vi "Main.vi"() -> ()   [LabVIEW 2026]
uses:
  3D utilities/3DS Models.ctl
  typedefs/System States.ctl
  typedefs/Render States.ctl
  <vilib>/picture/3D Picture Control/Old 3D Toolkit.llb/model.ctl
  <vilib>/picture/3D Picture Control/Old 3D Toolkit.llb/point3f.ctl
  <vilib>/picture/3D Picture Control/Old 3D Toolkit.llb/VertexMode.ctl
  <vilib>/vision/Image Controls.llb/IMAQ Image.ctl
  XRay Cabinet/XRay Cabinet.lvclass
  C:/Users/Andrey/Desktop/XRaySimulatorLV/XRay Scene/XRay Scene.lvclass
  XRay Beam/XRay Beam.lvclass
  XRay CArm/XRay CArm.lvclass
  XRay Part Sample/XRay Part Sample.lvclass
  XRay Table/XRay Table.lvclass
  XRay Beam/XRay Beam.lvclass/XRay Beam.ctl
  XRay Part Sample/XRay Part Sample.lvclass/XRay Part Sample.ctl
  XRay Table/XRay Table.lvclass/XRay Table.ctl
  <vilib>/Analysis/coordinate.llb/3D Cartesian Coordinate Rotation (Euler) (Scalar).vi
  67ea9b9f-5008-4843-b879-74d7c71b0f0c.vi
  XRay Axis Rails/XRay Axis Rails.lvclass
  <vilib>/picture/3D Picture Control/Object/Create Object.vi
  <vilib>/picture/3D Picture Control/Object/Create Object (name).vi
  <vilib>/picture/3D Picture Control/Geometries/Create 3D Axis.vi
  <vilib>/picture/3D Picture Control/Object/Add Object.vi
  <vilib>/picture/3D Picture Control/Object/Add Object (no reference).vi
  XRay Scene/XRay Scene.lvclass
  <vilib>/vision/NI_Vision_Development_Module.lvlib
  <vilib>/Analysis/NI_AALPro.lvlib
  3D utilities/3D utilities.lvlib
  <vilib>/picture/3D Picture Control/NI_Old 3D Toolkit.lvlib
  LV_3D_Util64.dll
panel:
  in  "Link to Z":bool
  in  "Mode":T1(ring)=enum."Wireframe"
  in  "High Res Render":bool
  in  "Play Button":bool
  in  "Reset":bool
  out "Render":bool
  in  "stop":bool
  in  "Part Angle":dbl(knob) caption="Part\nAngle"
  out "2D Image":T2(plugin-control)
  in  "Model":T3=enum."NI Bottle"
  in  "FDD":sgl(slide)=11.031496 scale=1.0..15.0
  in  "DDA SIZE":sgl(slide)=2.003937 scale=1.0..4.0
  out "Size":i32=1240
  out "Time, ms":dbl=63.153
  out "Max Thickness":sgl=0.5478592
  in  "Y Position":dbl(slide)=7.0 scale=1.0..12.0
  in  "X Position":dbl(slide)=0.5 scale=-2.0..2.0
  in  "C Arm Angle":dbl(knob) caption="C-Arm\nAngle" scale=90.0..-90.0
  in  "Z position":sgl(slide)=4.0 scale=0.0..10.0
  out "3D Picture":refnum<vi>(3d-picture)
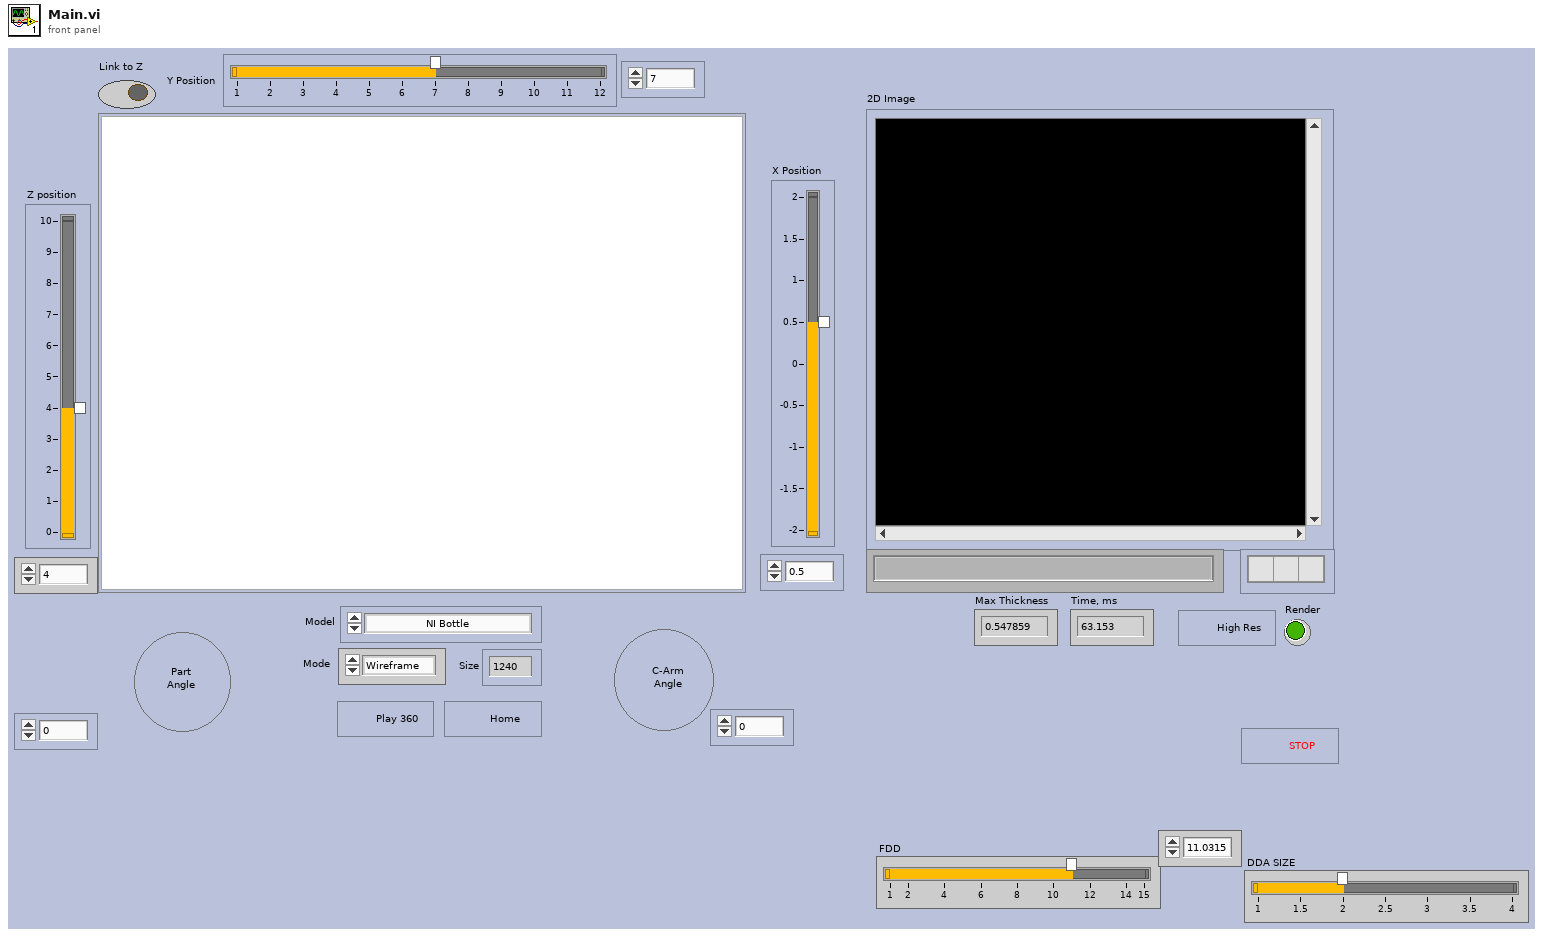
[diagram p1: front panel]
types:
  T1 = enum16{"Inherit Value", "Points", "Wireframe", "Polygons"}
  T2 = typedef "IMAQ Image.ctl" = refnum<image>
  T3 = typedef "3DS Models.ctl" = enum16{"ASTM E2597 Step Wedge", "NI Bottle", "Utah Teapot", "Utah Teapot (Low Res)", "My Cube", "Tree", "Tree 2", "FreeCAD Sample", "Schenkel", "Bunny", "Corona Virus", "Corona Virus (Low Res)", "Offset"}
  T4 = typedef "Render States.ctl" = enum16{"Init", "Create Model", "Move Model", "Render Model", "Render Model (High Res)", "Waiting for Command"}
  T5 = typedef "System States.ctl" = enum16{"Init", "Render", "Waiting for Notification", "Move", "Move 2D Model", "Close and reopen Model", "Quit"}
  T6 = typedef "NI_3D Picture Control.lvlib/NI_Old 3D Toolkit.lvlib/point3f.ctl" = cluster{"x":sgl, "y":sgl, "z":sgl}
  T7 = enum32{"Linear", "Log", "Exp", "Square", "Square root", "Power X", "Power 1/X"}
  T8 = cluster{"XRay Cabinet":refnum<class "XRay Cabinet.lvclass">, "XRay Beam":refnum<class "XRay Beam.lvclass">, "XRay CArm":refnum<class "XRay CArm.lvclass">, "XRay Part Sample":refnum<class "XRay Part Sample.lvclass">, "XRay Table":refnum<class "XRay Table.lvclass">}
  T9 = typedef "Image Type" = u32
  T10 = typedef "NI_3D Picture Control.lvlib/NI_Old 3D Toolkit.lvlib/model.ctl" = cluster{"VertexList":T6[], "FaceList":cluster{"v1":i32, "v2":i32, "v3":i32}[], "NormalList":T6[], "Mode":T11}
  T11 = typedef "NI_3D Picture Control.lvlib/NI_Old 3D Toolkit.lvlib/VertexMode.ctl" = enum16{"GL_POINTS", "GL_LINES", "GL_LINE_LOOP", "GL_LINE_STRIP", "GL_TRIANGLES", "GL_TRIANGLE_STRIP", "GL_TRIANGLE_FAN", "GL_QUADS", "GL_QUAD_STRIP", "GL_POLYGON"}
  T12 = cluster{"Model":T10, "Rendered Image":T2, "Processed Image":T2, "Vertex":T6[], "FaceList":cluster{"v1":i32, "v2":i32, "v3":i32}[]}
  T13 = cluster{"histogram":u32[], "Minimal Value":sgl, "Maximal Value":sgl, "Starting Value":sgl, "Interval Width":sgl, "Mean Value":sgl, "Standard  Variation":sgl, "Area (pixels)":i32}
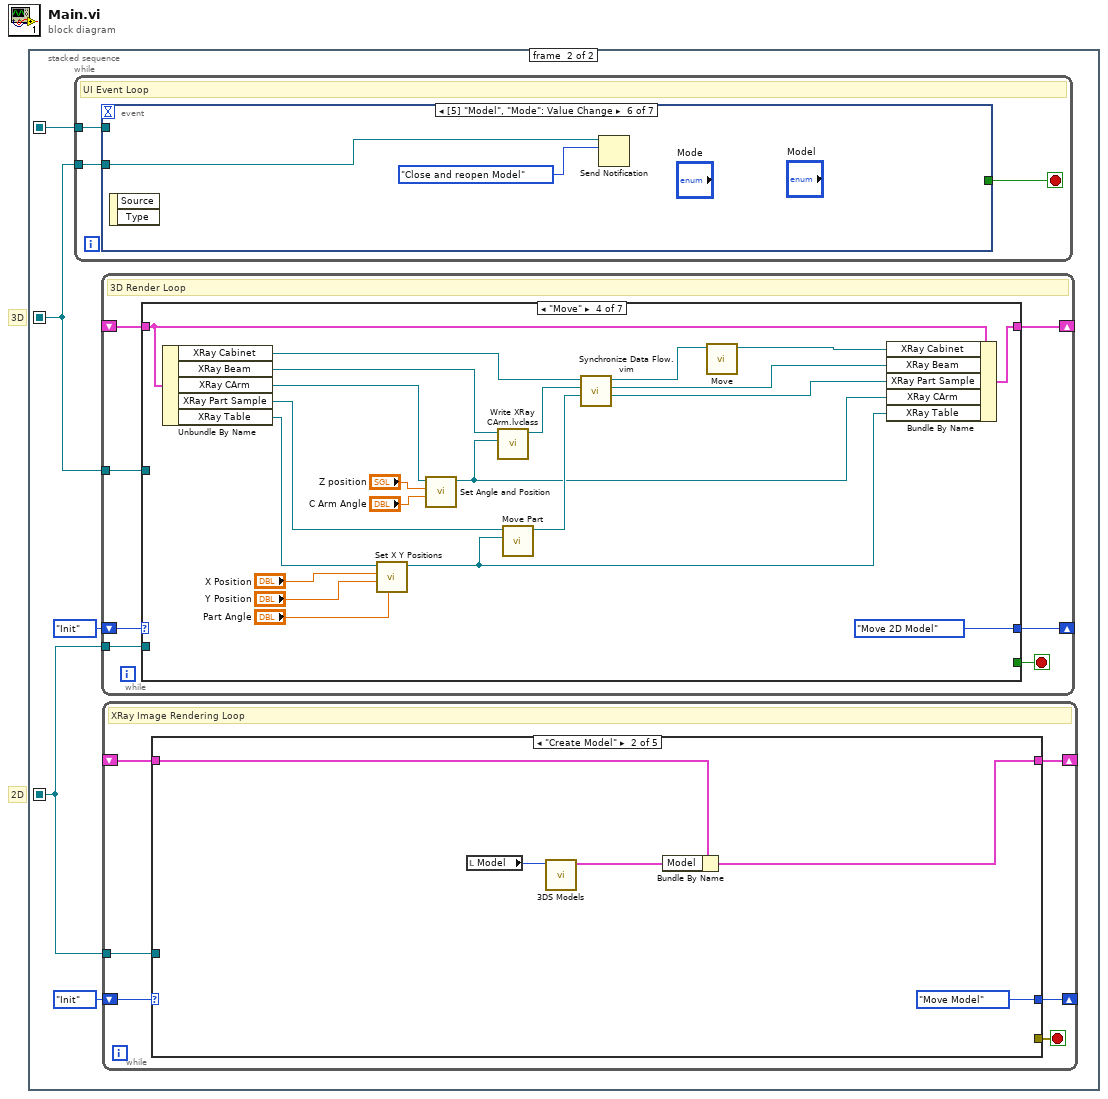
[diagram p0: block diagram]
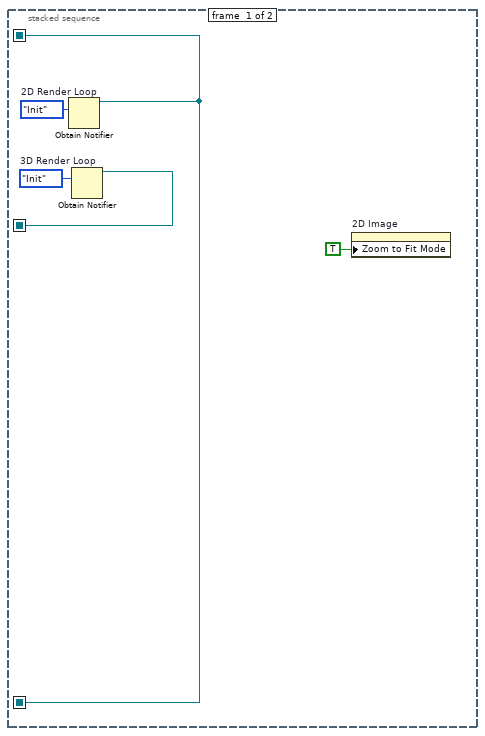
[diagram p2: hidden frame]
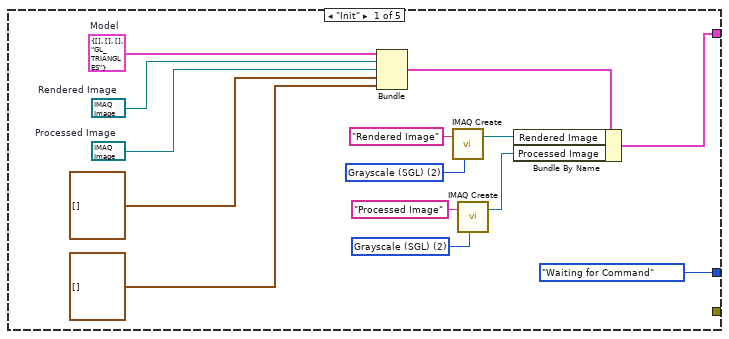
[diagram p3: hidden frame]
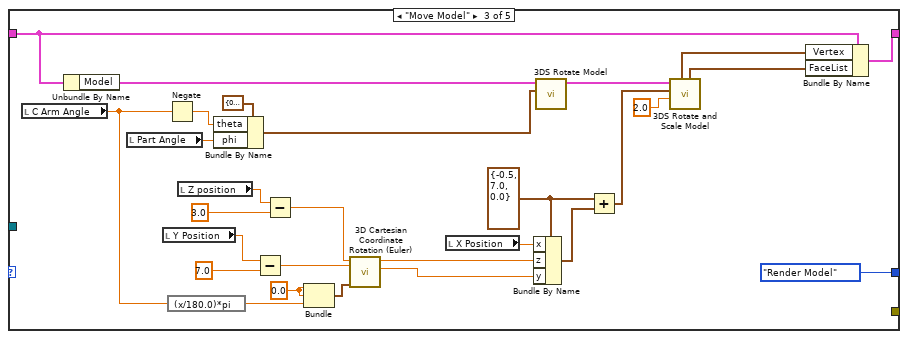
[diagram p4: hidden frame]
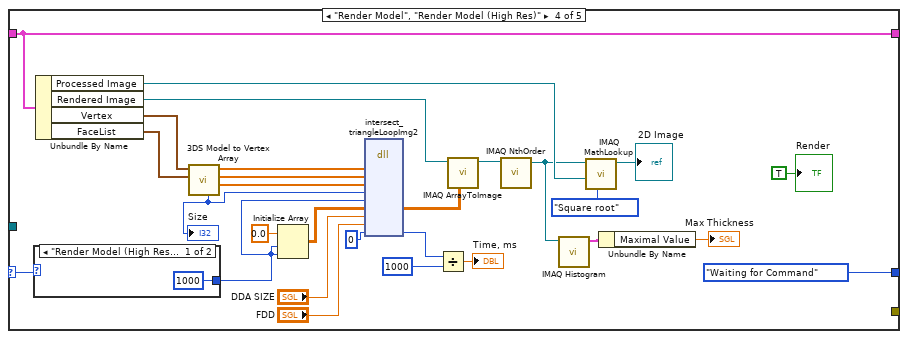
[diagram p5: hidden frame]
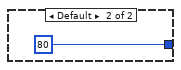
[diagram p6: hidden frame]
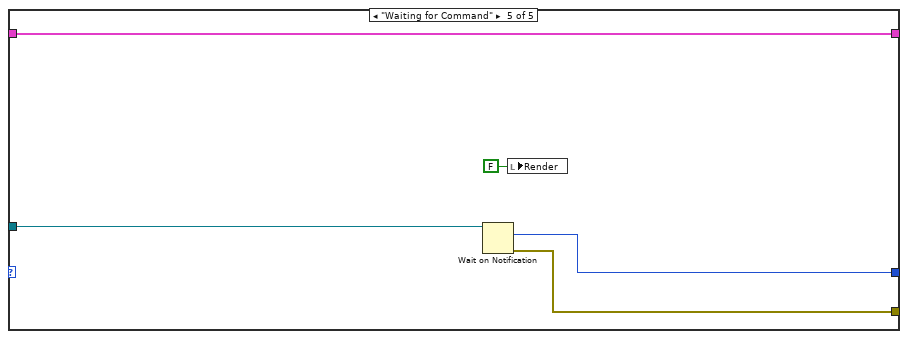
[diagram p7: hidden frame]
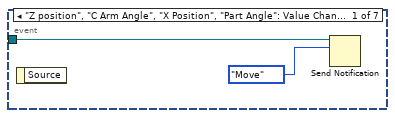
[diagram p8: hidden frame]
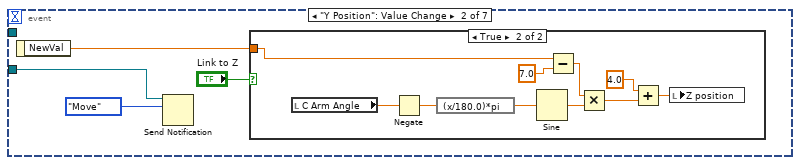
[diagram p9: hidden frame]
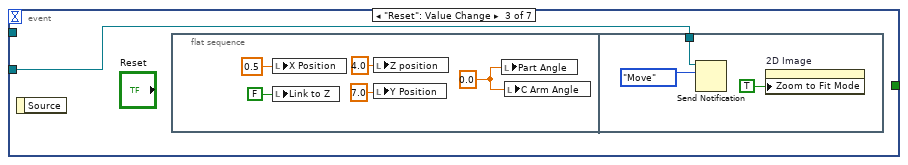
[diagram p11: hidden frame]
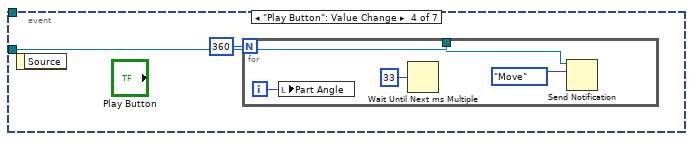
[diagram p12: hidden frame]
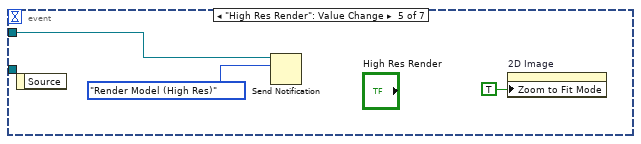
[diagram p13: hidden frame]
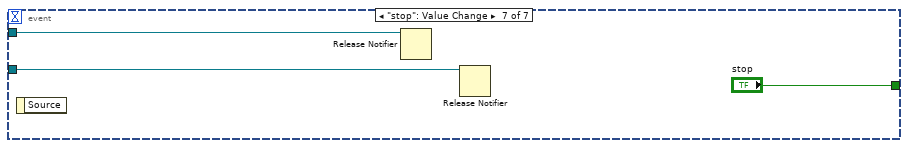
[diagram p14: hidden frame]
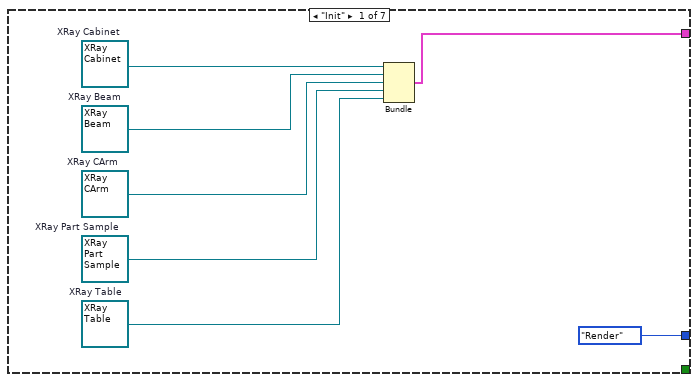
[diagram p15: hidden frame]
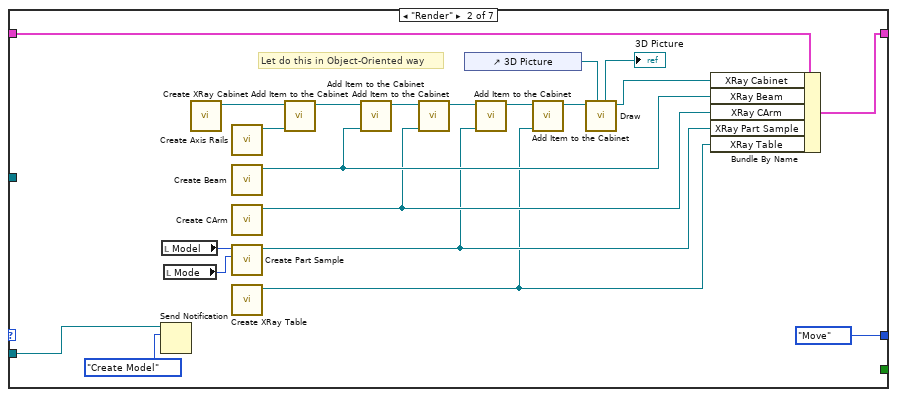
[diagram p16: hidden frame]
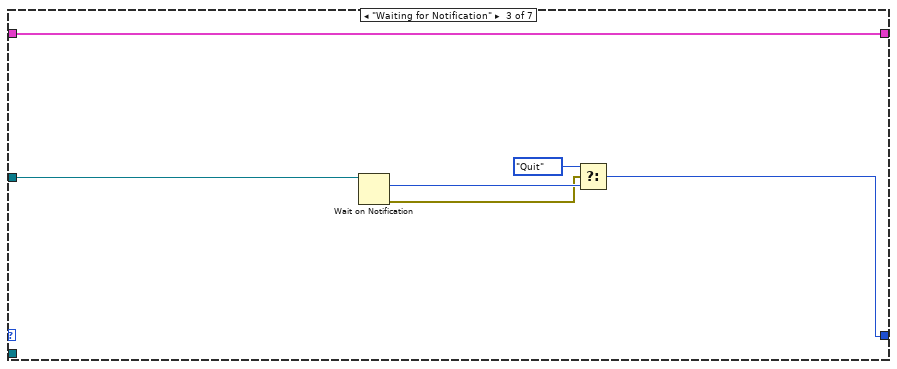
[diagram p17: hidden frame]
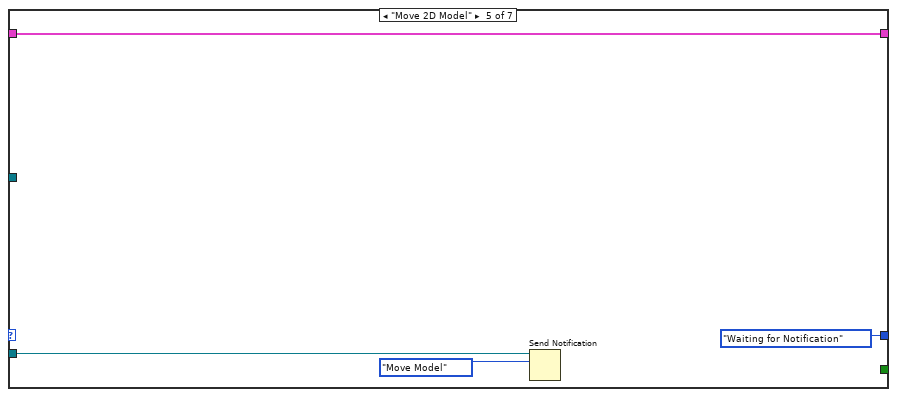
[diagram p18: hidden frame]
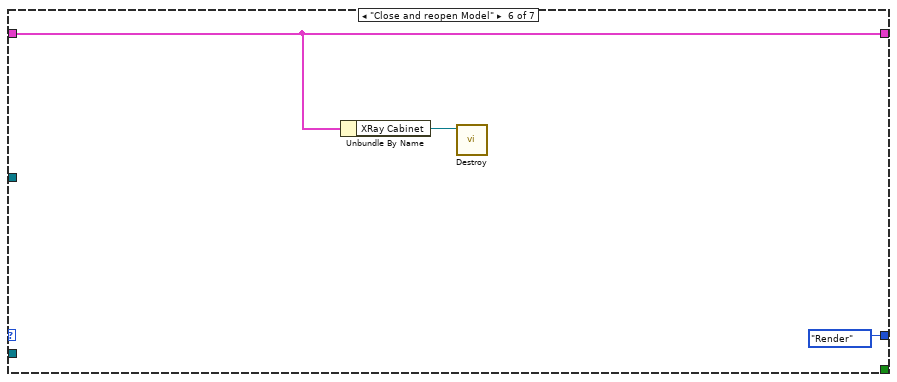
[diagram p19: hidden frame]
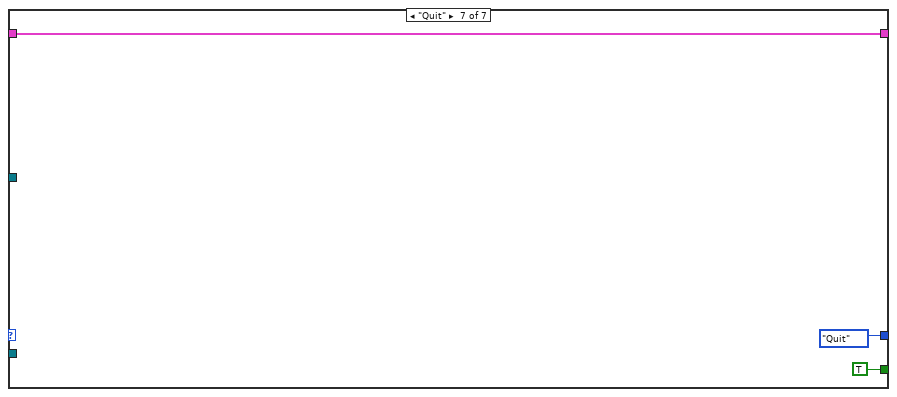
[diagram p20: hidden frame]
diagram:
  # "3D"
  # "2D"
  n1 = stacked-sequence {
    seq-local: [w3 _] -> [_ w6]
    seq-local: [w1 _] -> [_ w8]
    seq-local: [w1 _] -> [_ w7]
    frame #0 {
      w5 = Render_States."Init"  # 2D Render Loop
      w4 = System_States."Init"  # 3D Render Loop
      n2 = Obtain Notifier(notification data type=w5) -> (notifier out=w1:refnum<notifier>)  [unwired: 2 in, 3 out]
      n3 = Obtain Notifier(notification data type=w4) -> (notifier out=w3:refnum<notifier>)  [unwired: 2 in, 3 out]
      n4 = property on="2D Image" class="ImageControl"("Zoom to Fit Mode"=TRUE) -> ()  [unwired: 2 in, 2 out]
    }
    frame #1 {
      n5 = while {
        tunnel: w7 -> [w100]
        tunnel: w6 -> [w99]
        stop <- w101 stop-if-true
        # "UI Event Loop"
        n6 = event shown="[5] \"Model\", \"Mode\": Value Change" {
          selector: _ -> [_ _ _ _ _ _ _]
          dyn-events: _ -> [_ _ _ _ _ _ _]
          timeout: _ -> [_ _ _ _ _ _ _]
          tunnel: w99 -> [w103 w106 w118 w127 _ w136 w139]
          tunnel: [_ _ _ _ _ _ "stop"] -> w101
          tunnel: w100 -> [_ _ _ _ w135 _ w138]
          event "Z position", "C Arm Angle", "X Position", "Part Angle": Value Change {
            n7 = event-data() -> ()  [unwired: 1 in, 1 out]
            n8 = Send Notification(notification=System_States."Move", notifier=w103) -> ()  [unwired: 1 in, 2 out]
          }
          event "Y Position": Value Change {
            n9 = event-data() -> ("NewVal"=w105:dbl)  [unwired: 1 in]
            n10 = Send Notification(notification=System_States."Move", notifier=w106) -> ()  [unwired: 1 in, 2 out]
            n11 = case shown="True" "Link to Z" {
              tunnel: w105 -> [_ w112]
              frame False {
              }
              frame True {
                n12 = local read "C Arm Angle"() -> (w115:dbl)
                n13 = Negate(x=w115) -> (-x=w114:dbl)
                n14 = expression code="(x/180.0)*pi" ("degrees to radians")(w114) -> (w113:dbl)
                n15 = Sine(x=w113) -> (sin(x)=w108:dbl)
                n16 = Subtract(x=w112, y=7.0) -> (x-y=w110:dbl)
                n17 = Multiply(x=w110, y=w108) -> (x*y=w109:dbl)
                n18 = Add(x=4.0, y=w109) -> (x+y=w116:dbl)
                n19 = local write "Z position"(w116) -> ()
              }
            }
          }
          event "Reset": Value Change {
            n20 = event-data() -> ()  [unwired: 1 in, 1 out]
            n21 = flat-sequence {
              tunnel: w118 -> [w126]
              frame #0 {
                w120 = 0.0 ("Part Angle")
                n22 = local write "X Position"(0.5 ("X Position")) -> ()
                n23 = local write "Link to Z"(FALSE ("Link to Z")) -> ()
                n24 = local write "Z position"(sgl 4.0 ("Z position")) -> ()
                n25 = local write "Y Position"(7.0 ("Y Position")) -> ()
                n26 = local write "Part Angle"(w120) -> ()
                n27 = local write "C Arm Angle"(w120) -> ()
              }
              frame #1 {
                n28 = Send Notification(notification=System_States."Move", notifier=w126) -> ()  [unwired: 1 in, 2 out]
                n29 = property on="2D Image" class="ImageControl"("Zoom to Fit Mode"=TRUE) -> ()  [unwired: 2 in, 2 out]
              }
            }
          }
          event "Play Button": Value Change {
            n30 = event-data() -> ()  [unwired: 1 in, 1 out]
            n31 = for {
              N: 360 -> [_]
              tunnel: w127 -> [w130]
              i -> [w132]
              n32 = local write "Part Angle"(w132) -> ()
              n33 = Wait Until Next ms Multiple(millisecond multiple=u32 33) -> ()  [unwired: 1 out]
              n34 = Send Notification(notification=System_States."Move", notifier=w130) -> ()  [unwired: 1 in, 2 out]
            }
          }
          event "High Res Render": Value Change {
            n35 = event-data() -> ()  [unwired: 1 in, 1 out]
            n36 = Send Notification(notification=Render_States."Render Model (High Res)", notifier=w135) -> ()  [unwired: 1 in, 2 out]
            n37 = property on="2D Image" class="ImageControl"("Zoom to Fit Mode"=TRUE) -> ()  [unwired: 2 in, 2 out]
          }
          event "Mode": Value Change {
            n38 = event-data() -> ()  [unwired: 1 in, 2 out]
            n39 = Send Notification(notification=System_States."Close and reopen Model", notifier=w136) -> ()  [unwired: 1 in, 2 out]
          }
          event "stop": Value Change {
            n40 = event-data() -> ()  [unwired: 1 in, 1 out]
            n41 = Release Notifier(notifier=w138) -> ()  [unwired: 1 in, 4 out]
            n42 = Release Notifier(notifier=w139) -> ()  [unwired: 1 in, 4 out]
          }
        }
      }
      n43 = while {
        shift-right: [w146] -> _
        shift-left: System_States."Init" -> [w147]
        shift-right: [w145] -> _
        shift-left: _ -> [w144]
        tunnel: w6 -> [w143]
        tunnel: w8 -> [w141]
        stop <- w142 stop-if-true
        # "3D Render Loop"
        n44 = case shown="\"Move\"" w147 {
          tunnel: [System_States."Render" System_States."Move" w177 System_States."Move 2D Model" System_States."Waiting for Notification" System_States."Render" System_States."Quit"] -> w146
          tunnel: [w148 w160 w181 w186 w203 w208 w210] -> w145
          tunnel: w144 -> [_ w166 w181 w190 w203 w208 w210]
          tunnel: w143 -> [_ _ w180 _ _ _ _]
          tunnel: [_ _ _ _ _ _ TRUE] -> w142
          tunnel: w141 -> [_ w157 _ _ w205 _ _]
          frame "Init" {
            w149 = refnum<class "XRay Table.lvclass"> refnum  # XRay Table
            w150 = refnum<class "XRay Part Sample.lvclass"> refnum  # XRay Part Sample
            w151 = refnum<class "XRay CArm.lvclass"> refnum  # XRay CArm
            w152 = refnum<class "XRay Beam.lvclass"> refnum  # XRay Beam
            w153 = refnum<class "XRay Cabinet.lvclass"> refnum  # XRay Cabinet
            n45 = Bundle("XRay Cabinet"=w153, "XRay Beam"=w152, "XRay CArm"=w151, "XRay Part Sample"=w150, "XRay Table"=w149) -> (w148:T8)  [unwired: 1 in]
          }
          frame "Render" {
            # "Let do this in Object-Oriented way"
            n46 = Send Notification(notification=Render_States."Create Model", notifier=w157) -> ()  [unwired: 1 in, 2 out]
            n47 = local read "Model"() -> (w158:T3)
            n48 = local read "Mode"() -> (w155:T1)
            n49 = call "Create XRay Cabinet.vi"() -> ("XRay Cabinet out"=w170:refnum<class "XRay Cabinet.lvclass">)  [unwired: 10 in, 1 out]
            n50 = call "Create Axis Rails.vi"() -> ("XRay Axis Rails out"=w168:refnum<class "XRay Axis Rails.lvclass">)  [unwired: 10 in, 1 out]
            n51 = call "Create Beam.vi"() -> ("XRay Beam out"=w164:refnum<class "XRay Beam.lvclass">)  [unwired: 10 in, 1 out]
            n52 = call "Create CArm.vi"() -> ("XRay CArm out"=w163:refnum<class "XRay CArm.lvclass">)  [unwired: 10 in, 1 out]
            n53 = call "Create Part Sample.vi"("Draw Style:Mode"=w155, "Model"=w158) -> ("XRay Part Sample out"=w162:refnum<class "XRay Part Sample.lvclass">)  [unwired: 8 in, 1 out]
            n54 = call "Create XRay Table.vi"() -> ("XRay Table out"=w161:refnum<class "XRay Table.lvclass">)  [unwired: 10 in, 1 out]
            n55 = call "Add Item to the Cabinet.vi"("Object"=w168, "XRay Cabinet In"=w170) -> ("XRay Cabinet Out"=w167:refnum<class "XRay Cabinet.lvclass">)  [unwired: 9 in]
            n56 = call "Add Item to the Cabinet.vi"("Object"=w164, "XRay Cabinet In"=w167) -> ("XRay Cabinet Out"=w171:refnum<class "XRay Cabinet.lvclass">)  [unwired: 9 in]
            n57 = call "Add Item to the Cabinet.vi"("Object"=w163, "XRay Cabinet In"=w171) -> ("XRay Cabinet Out"=w173:refnum<class "XRay Cabinet.lvclass">)  [unwired: 9 in]
            n58 = control-ref of="3D Picture"() -> (w169:refnum<vi>)
            n59 = call "Add Item to the Cabinet.vi"("Object"=w162, "XRay Cabinet In"=w173) -> ("XRay Cabinet Out"=w174:refnum<class "XRay Cabinet.lvclass">)  [unwired: 9 in]
            n60 = call "Add Item to the Cabinet.vi"("Object"=w161, "XRay Cabinet In"=w174) -> ("XRay Cabinet Out"=w172:refnum<class "XRay Cabinet.lvclass">)  [unwired: 9 in]
            n61 = call "Draw.vi"("3D Picture"=w169, "XRay Scene in"=w172) -> ("XRay Scene out"=w165:refnum<class "XRay Cabinet.lvclass">, "Scene Object"=→"3D Picture":refnum<vi>)  [unwired: 7 in, 1 out]
            n62 = Bundle By Name(cluster=w166, "XRay Cabinet"=w165, "XRay Beam"=w164, "XRay CArm"=w163, "XRay Part Sample"=w162, "XRay Table"=w161) -> (w160:T8)
          }
          frame "Waiting for Notification" {
            n63 = Wait on Notification(notifier=w180) -> (notification=w179:T5, error out=w178:errorcluster)  [unwired: 1 in, 4 out]
            n64 = Select(t=System_States."Quit", s=w178, f=w179) -> (s? t:f=w177:T5)
          }
          frame "Move" {
            n65 = Unbundle By Name(w190) -> ("XRay Cabinet"=w195:refnum<class "XRay Cabinet.lvclass">, "XRay Beam"=w194:refnum<class "XRay Beam.lvclass">, "XRay CArm"=w193:refnum<class "XRay CArm.lvclass">, "XRay Part Sample"=w192:refnum<class "XRay Part Sample.lvclass">, "XRay Table"=w191:refnum<class "XRay Table.lvclass">)
            n66 = call "Set X Y Positions.vi"("Table Rotation"="Part Angle", "Y Position"="Y Position", "X Position"="X Position", "XRay Table in"=w191) -> ("XRay Table out"=w183:refnum<class "XRay Table.lvclass">)  [unwired: 6 in, 1 out]
            n67 = call-dynamic "Set Angle and Position.vi"("Angle"="C Arm Angle", "Z"="Z position", "XRay CArm in"=w193) -> ("XRay CArm out"=w184:refnum<class "XRay CArm.lvclass">)  [unwired: 7 in, 1 out]
            n68 = call "Write XRay CArm.lvclass.vi"("XRay CArm.lvclass"=w184, "XRay Beam in"=w194) -> ("XRay Beam out"=w197:refnum<class "XRay Beam.lvclass">)  [unwired: 8 in, 1 out]
            n69 = call "Move Part.vi"("XRay Table.lvclass"=w183, "XRay Part Sample in"=w192) -> ("XRay Part Sample out"=w187:refnum<class "XRay Part Sample.lvclass">)  [unwired: 8 in, 1 out]
            n70 = call "Synchronize Data Flow.vim"("input 3"=w187, "input 2"=w197, "input 1"=w195) -> ("output 3"=w185:refnum<class "XRay Part Sample.lvclass">, "output 2"=w188:refnum<class "XRay Beam.lvclass">, "output 1"=w198:refnum<class "XRay Cabinet.lvclass">)  [unwired: 1 in, 1 out]
            n71 = call-dynamic "Move.vi"("XRay Scene in"=w198) -> ("XRay Scene out"=w189:refnum<class "XRay Cabinet.lvclass">)  [unwired: 8 in, 2 out]
            n72 = Bundle By Name(cluster=w190, "XRay Cabinet"=w189, "XRay Beam"=w188, "XRay Part Sample"=w185, "XRay CArm"=w184, "XRay Table"=w183) -> (w186:T8)
          }
          frame "Move 2D Model" {
            n73 = Send Notification(notification=Render_States."Move Model", notifier=w205) -> ()  [unwired: 1 in, 2 out]
          }
          frame "Close and reopen Model" {
            n74 = Unbundle By Name(w208) -> ("XRay Cabinet"=w207:refnum<class "XRay Cabinet.lvclass">)
            n75 = call-dynamic "Destroy.vi"("XRay Cabinet in"=w207) -> ()  [unwired: 9 in, 2 out]
          }
          frame "Quit" {
          }
        }
      }
      n76 = while {
        shift-right: [w13] -> _
        shift-left: Render_States."Init" -> [w16]
        shift-right: [w15] -> _
        shift-left: _ -> [w14]
        tunnel: w8 -> [w12]
        stop <- w11 stop-if-true
        # "XRay Image Rendering Loop"
        n77 = case shown="\"Create Model\"" w16 {
          selector: w16 -> [_ _ _ w68 _]
          tunnel: [w20 w34 w44 w72 w98] -> w15
          tunnel: w14 -> [_ w35 w45 w72 w98]
          tunnel: [Render_States."Waiting for Command" Render_States."Move Model" Render_States."Render Model" Render_States."Waiting for Command" w96] -> w13
          tunnel: w12 -> [_ _ _ _ w97]
          tunnel: [_ _ _ _ w95] -> w11
          frame "Init" {
            w21 = T9 2 items=["Grayscale (U8)", "Grayscale (I16)", "Grayscale (SGL)", "Complex (CSG)", "RGB (U32)", "HSL (U32)", "RGB (U64)", "Grayscale (U16)"] ("Image Type")
            w25 = T9 2 items=["Grayscale (U8)", "Grayscale (I16)", "Grayscale (SGL)", "Complex (CSG)", "RGB (U32)", "HSL (U32)", "RGB (U64)", "Grayscale (U16)"] ("Image Type")
            w28 = T2 refnum  # Processed Image
            w29 = T2 refnum  # Rendered Image
            w30 = T10 {"VertexList"=[], "FaceList"=[], "NormalList"=[], "Mode"=enum."GL_TRIANGLES"}  # Model
            n78 = Bundle("Model"=w30, "Rendered Image"=w29, "Processed Image"=w28, "Vertex"=T6[] [], "FaceList"=cluster{"v1":i32, "v2":i32, "v3":i32}[] []) -> (w27:T12)  [unwired: 1 in]
            n79 = call "IMAQ Create"("Image Name"="Rendered Image", "Image Type"=w25) -> ("New Image"=w24:T2)  [unwired: 3 in, 1 out]
            n80 = call "IMAQ Create"("Image Name"="Processed Image", "Image Type"=w21) -> ("New Image"=w22:T2)  [unwired: 3 in, 1 out]
            n81 = Bundle By Name(cluster=w27, "Rendered Image"=w24, "Processed Image"=w22) -> (w20:T12)
          }
          frame "Create Model" {
            n82 = local read "Model"() -> (w31:T3)
            n83 = call "3DS Models.vi"("Model"=w31) -> ("Model Out"=w32:T10)  [unwired: 10 in]
            n84 = Bundle By Name(cluster=w35, "Model"=w32) -> (w34:T12)
          }
          frame "Move Model" {
            w41 = T6 {"x"=-0.5, "y"=7.0, "z"=0.0} ("point3f - SHIFT")
            w52 = 0.0 ("x/y")
            n85 = local read "C Arm Angle"() -> (w36:dbl)
            n86 = Unbundle By Name(w45) -> ("Model"=w48:T10)
            n87 = local read "Part Angle"() -> (w63:dbl)
            n88 = local read "Y Position"() -> (w58:dbl)
            n89 = Negate(x=w36) -> (-x=w59:dbl)
            n90 = expression code="(x/180.0)*pi" ("degrees to radians")(w36) -> (w42:dbl)
            n91 = local read "Z position"() -> (w57:sgl)
            n92 = Bundle By Name(cluster=cluster{"phi":dbl, "theta":dbl, "psi":dbl} {"phi"=0.0, "theta"=0.0, "psi"=1.0} ("Euler Angles"), "theta"=w59, "phi"=w63) -> (w55:cluster{"phi":dbl, "theta":dbl, "psi":dbl})
            n93 = Subtract(x=w58, y=7.0) -> (x-y=w60:dbl)
            n94 = Subtract(x=w57, y=3.0) -> (x-y=w61:dbl)
            n95 = Bundle("x/y"=w52, "x/y"=w52, "C Arm Angle"=w42) -> (w62:cluster{"x/y":dbl, "x/y":dbl, "C Arm Angle":dbl})  [unwired: 1 in]
            n96 = call-poly <vilib>:"3D Cartesian Coordinate Rotation (Euler).vi"("Euler Angles"=w62, "y"=w60, "x"=w61) -> ("y out"=w38:dbl, "x out"=w39:dbl)  [unwired: 5 in, 2 out]
            n97 = local read "X Position"() -> (w40:dbl)
            n98 = Bundle By Name(cluster=w41, "x"=w40, "z"=w39, "y"=w38) -> (w37:T6)
            n99 = call "3DS Rotate Model.vi"("Euler Angles"=w55, "model in"=w48) -> ("model out"=w54:T10)  [unwired: 9 in]
            n100 = Add(x=w41, y=w37) -> (x+y=w56:T6)
            n101 = call "3DS Rotate and Scale Model.vi"("scale"=sgl 2.0, "point3f - SHIFT"=w56, "Object In"=w54) -> ("FaceList"=w46:cluster{"v1":i32, "v2":i32, "v3":i32}[], "Vertex"=w47:T6[])  [unwired: 5 in, 2 out]
            n102 = Bundle By Name(cluster=w45, "Vertex"=w47, "FaceList"=w46) -> (w44:T12)
          }
          frame "Render Model", "Render Model (High Res)" {
            n103 = case shown="\"Render Model (High Res)\"" w68 {
              tunnel: [1000 ("IMAGE SIZE") 80 ("IMAGE SIZE")] -> w67
              frame "Render Model (High Res)" {
              }
              frame Default {
              }
            }
            n104 = Unbundle By Name(w72) -> ("Processed Image"=w66:T2, "Rendered Image"=w70:T2, "Vertex"=w74:T6[], "FaceList"=w73:cluster{"v1":i32, "v2":i32, "v3":i32}[])
            n105 = call "3DS Model to Vertex Array.vi"("FaceList"=w73, "Array"=w74) -> ("point3f 2"=w84:sgl[], "point3f 3"=w83:sgl[], "point3f"=w86:sgl[], "Count"=w87:i32)  [unwired: 6 in]
            "Size" <- w87
            n106 = Initialize Array(sgl 0.0 ("element"), w67, w67) -> (w85:sgl[][])
            n107 = dll-call lib="C:/Users/Andrey/Desktop/XRaySimulatorLV/LV_3D_Util*.*" fn="intersect_triangleLoopImg2" ("LV_3D_Util.dll:\nintersect_\ntriangleL\noopImg2")("vert0"=w86, "vert1"=w83, "vert2"=w84, "MeshSize"=w87, "ImageSize"=w67, "image"=w85, "DetectorSize"="DDA SIZE", "FDD"="FDD", "Execution Time"=u64 0) -> ("image"=w79:sgl[][], "Execution Time"=w88:u64)  [unwired: 11 in, 2 out]
            n108 = Divide(x=w88, y=u64 1000) -> (x/y=→"Time, ms":dbl)
            n109 = call "IMAQ ArrayToImage"("Image Pixels (Float)"=w79, "Image"=w70) -> ("Image Out"=w80:T2)  [unwired: 8 in, 1 out]
            n110 = call "IMAQ NthOrder"("Image Src"=w80) -> ("Image Dst Out"=w65:T2)  [unwired: 6 in, 1 out]
            n111 = call "IMAQ Histogram"("Image"=w65) -> ("Histogram Report"=w90:T13)  [unwired: 9 in, 1 out]
            n112 = call "IMAQ MathLookup"("Operator"=T7."Square root", "Image Dst"=w66, "Image Src"=w65) -> ("Image Dst Out"=→"2D Image":T2)  [unwired: 7 in, 1 out]
            n113 = Unbundle By Name(w90) -> ("Maximal Value"=→"Max Thickness":sgl)
            "Render" <- TRUE ("Render")
          }
          frame "Waiting for Command" {
            n114 = Wait on Notification(notifier=w97) -> (notification=w96:T4, error out=w95:errorcluster)  [unwired: 1 in, 4 out]
            n115 = local write "Render"(FALSE ("Render")) -> ()
          }
        }
      }
    }
  }
